vi "SetCellColor.vi"(11 "Sensor Info":T1) -> (3 "Color":u32)   [LabVIEW 2018, in "HealthCheck.lvclass"]
uses:
  HealthCheck.lvclass
  DataEntry_TypeDef.ctl
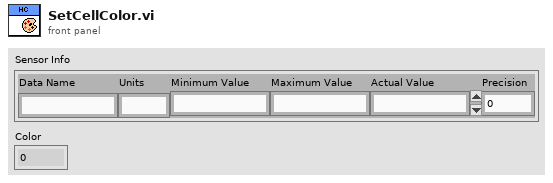
[diagram p1: front panel]
types:
  T1 = typedef "HealthCheck.lvclass/DataEntry_TypeDef.ctl" = cluster{"Data Name":string, "Units":string, "Minimum Value":string, "Maximum Value":string, "Actual Value":string, "Precision":i16}
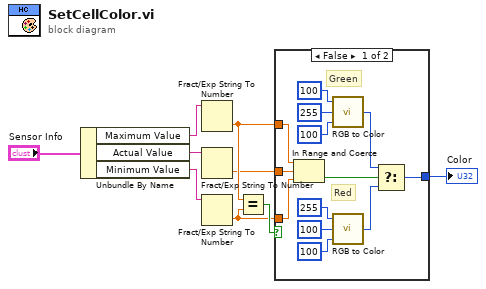
[diagram p0: block diagram]
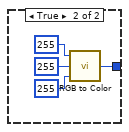
[diagram p2: hidden frame]
diagram:
  n1 = Unbundle By Name("Sensor Info") -> ("Maximum Value"=w4:string, "Actual Value"=w3:string, "Minimum Value"=w2:string)
  n2 = Fract/Exp String To Number(string=w4) -> (number=w7:dbl)  [unwired: 3 in, 1 out]
  n3 = Fract/Exp String To Number(string=w3) -> (number=w6:dbl)  [unwired: 3 in, 1 out]
  n4 = Fract/Exp String To Number(string=w2) -> (number=w8:dbl)  [unwired: 3 in, 1 out]
  n5 = Equal?(x=w7, y=w8) -> (x = y?=w9:bool)
  n6 = case shown="False" w9 {
    tunnel: [w11 w23] -> w1
    tunnel: w6 -> [w22 _]
    tunnel: w7 -> [w21 _]
    tunnel: w8 -> [w20 _]
    frame False {
      # "Red"
      # "Green"
      n7 = In Range and Coerce(upper limit=w21, x=w22, lower limit=w20) -> (In Range?=w12:bool)  [unwired: 1 out]
      n8 = call <vilib>:"RGB to Color.vi"("B"=u8 100, "G"=u8 255, "R"=u8 100) -> ("Color"=w10:u32)
      n9 = call <vilib>:"RGB to Color.vi"("B"=u8 100, "G"=u8 100, "R"=u8 255) -> ("Color"=w19:u32)
      n10 = Select(t=w10, s=w12, f=w19) -> (s? t:f=w11:u32)
    }
    frame True {
      n11 = call <vilib>:"RGB to Color.vi"("B"=u8 255, "G"=u8 255, "R"=u8 255) -> ("Color"=w23:u32)
    }
  }
  "Color" <- w1
